vi "Subvi Email Settings.vi"() -> ()   [LabVIEW 2012]
uses:
  ProSCI Global.vi
panel:
  in  "AttachImage":bool
  in  "Carrier":string(combo)="@message.alltel.com"
  in  "Continue":bool
  in  "Cellphone Number":string
  in  "SMSMe":bool
  in  "NotifyNum":u32=5 min=5 max=10000 step=5
  in  "EmailMe":bool
  in  "CaseID":string
  # "Sequence Progress Notification"
  # "Notify through"
  # "Attach Image with Email"
  # "(* Texting may incur charges from your cellphone carrier)"
  # "sections"
  # "Notify Me on Completion and every"
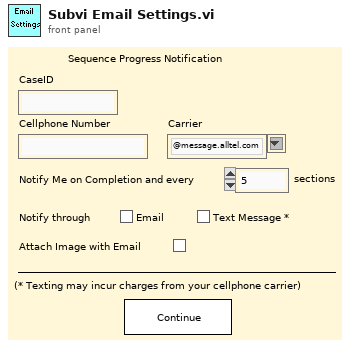
[diagram p1: front panel]
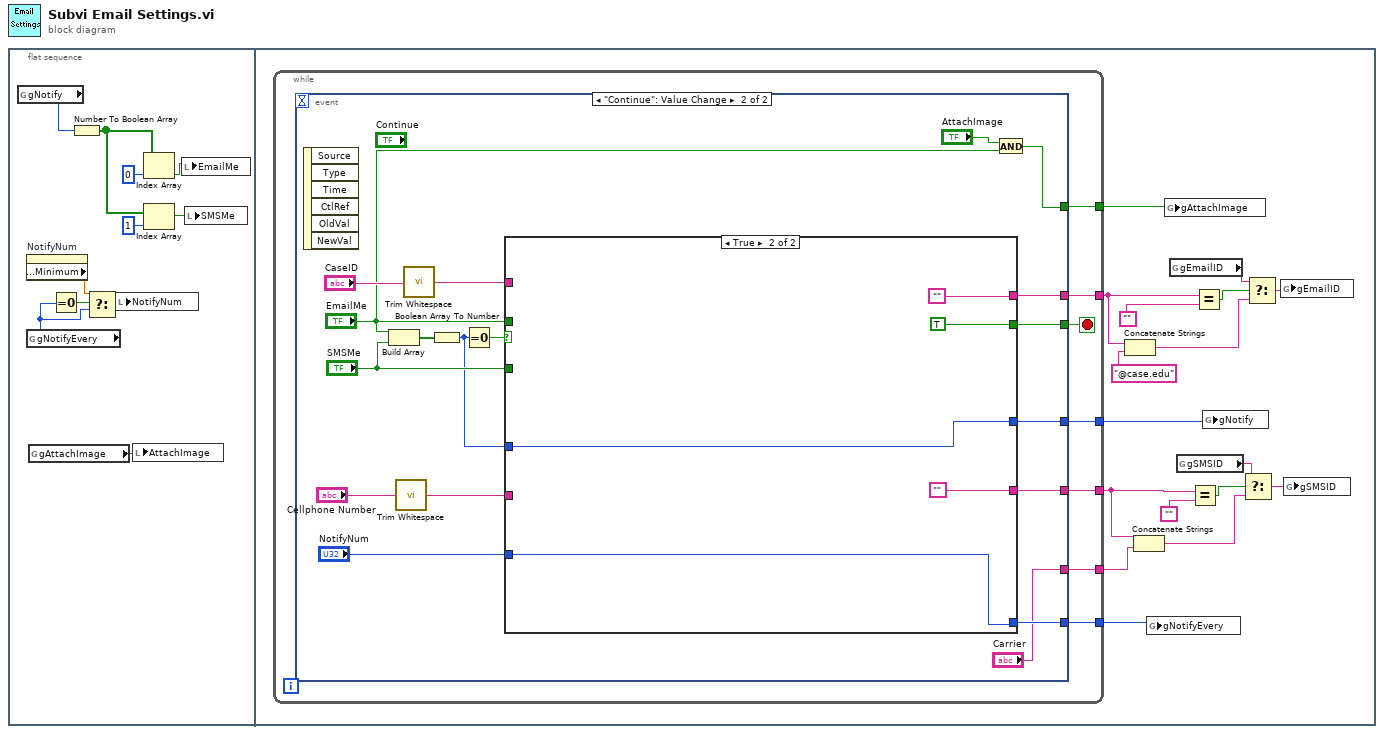
[diagram p0: block diagram]
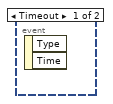
[diagram p2: hidden frame]
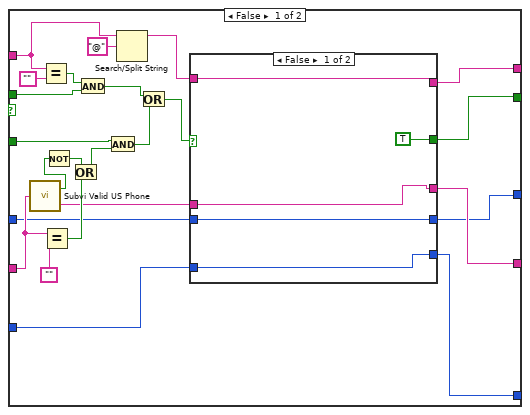
[diagram p3: hidden frame]
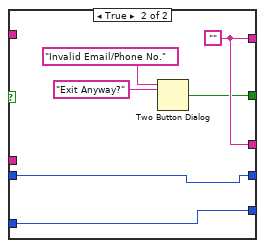
[diagram p4: hidden frame]
diagram:
  n1 = flat-sequence {
    frame #0 {
      n2 = global read "ProSCI Global.vi" "gNotify"() -> (w11:enum16{"None", "Email", "SMS", "Both"})
      n3 = property on="NotifyNum" class="DigNum (strict)"() -> ("Data Entry Limits:Minimum"=w1:dbl)  [unwired: 2 in, 2 out]
      n4 = global read "ProSCI Global.vi" "gNotifyEvery"() -> (w3:u32)
      n5 = global read "ProSCI Global.vi" "gAttachImage"() -> (w5:bool)
      n6 = Equal To 0?(x=w3) -> (x = 0?=w4:bool)
      n7 = Number To Boolean Array(number=w11) -> (Boolean array=w8:bool[])
      n8 = Select(t=w1, s=w4, f=w3) -> (s? t:f=w2:dbl)
      n9 = local write "NotifyNum"(w2) -> ()
      n10 = local write "AttachImage"(w5) -> ()
      n11 = Index Array(array=w8, index=0) -> (element=w7:bool)
      n12 = Index Array(array=w8, index=1) -> (element=w6:bool)
      n13 = local write "EmailMe"(w7) -> ()
      n14 = local write "SMSMe"(w6) -> ()
    }
    frame #1 {
      n15 = while {
        tunnel: [w34] -> w27
        tunnel: [w33] -> w22
        tunnel: [w32] -> w15
        tunnel: [w31] -> w14
        tunnel: [w30] -> w13
        tunnel: [w29] -> w12
        stop <- w35 stop-if-true
        n16 = event shown="[1] \"Continue\": Value Change" {
          selector: _ -> [_ _]
          dyn-events: _ -> [_ _]
          timeout: _ -> [_ _]
          tunnel: [_ w52] -> w35
          tunnel: [_ w48] -> w34
          tunnel: [_ w44] -> w33
          tunnel: [_ w43] -> w32
          tunnel: [_ w40] -> w31
          tunnel: [_ "Carrier"] -> w30
          tunnel: [_ w36] -> w29
          event Timeout {
            n17 = event-data() -> ()  [unwired: 3 out]
          }
          event "Continue": Value Change {
            n18 = event-data() -> ()  [unwired: 7 out]
            n19 = Build Array("EmailMe", "SMSMe") -> (w53:bool[])
            n20 = call <vilib>:"Trim Whitespace.vi"("string"="Cellphone Number") -> ("trimmed string"=w46:string)  [unwired: 1 in]
            n21 = call <vilib>:"Trim Whitespace.vi"("string"="CaseID") -> ("trimmed string"=w50:string)  [unwired: 1 in]
            n22 = Boolean Array To Number(Boolean array=w53) -> (number=w42:u32)
            n23 = Equal To 0?(x=w42) -> (x = 0?=w49:bool)
            n24 = case shown="True" w49 {
              tunnel: [w62 TRUE] -> w52
              tunnel: w50 -> [w76 _]
              tunnel: [w61 ""] -> w48
              tunnel: w46 -> [w70 _]
              tunnel: "EmailMe" -> [w72 _]
              tunnel: "SMSMe" -> [w71 _]
              tunnel: [w60 ""] -> w44
              tunnel: [w57 w89] -> w43
              tunnel: w42 -> [w56 w89]
              tunnel: "NotifyNum" -> [w55 w90]
              tunnel: [w54 w90] -> w40
              frame False {
                n25 = call "Subvi Valid US Phone.vi"("PhNumString"=w70) -> ("Is Valid"=w68:bool, "Valid Number"=w58:string)
                n26 = Equal?(x=w76, y="") -> (x = y?=w73:bool)
                n27 = Equal?(x=w70, y="") -> (x = y?=w67:bool)
                n28 = Not(x=w68) -> (.not. x?=w69:bool)
                n29 = Or(x=w69, y=w67) -> (x .or. y?=w66:bool)
                n30 = And(x=w73, y=w72) -> (x .and. y?=w65:bool)
                n31 = And(x=w71, y=w66) -> (x .and. y?=w64:bool)
                n32 = Search/Split String(string=w76, search string/char (-)="@") -> (substring before match=w59:string)  [unwired: 3 out]
                n33 = Or(x=w65, y=w64) -> (x .or. y?=w63:bool)
                n34 = case shown="False" w63 {
                  tunnel: [TRUE ("T button?") w85] -> w62
                  tunnel: [w81 w86] -> w61
                  tunnel: [w80 w86] -> w60
                  tunnel: w59 -> [w81 _]
                  tunnel: w58 -> [w80 _]
                  tunnel: [w79 w84] -> w57
                  tunnel: w56 -> [w79 w84]
                  tunnel: w55 -> [w78 w83]
                  tunnel: [w78 w83] -> w54
                  frame False {
                  }
                  frame True {
                    w86 = ""
                    n35 = Two Button Dialog(message="Invalid Email/Phone No.", 2:"Exit Anyway?" ("T button name (\"OK\")")) -> (T button?=w85:bool)  [unwired: 1 out]
                  }
                }
              }
              frame True {
              }
            }
            n36 = And(x="AttachImage", y="EmailMe") -> (x .and. y?=w36:bool)
          }
        }
      }
      n37 = Concatenate Strings(w27, "@case.edu") -> (w25:string)
      n38 = Concatenate Strings(w22, w13) -> (w23:string)
      n39 = global write "ProSCI Global.vi" "gNotifyEvery"(w14) -> ()
      n40 = global write "ProSCI Global.vi" "gAttachImage"(w12) -> ()
      n41 = global read "ProSCI Global.vi" "gEmailID"() -> (w17:string)
      n42 = global read "ProSCI Global.vi" "gSMSID"() -> (w16:string)
      n43 = Equal?(x=w22, y="") -> (x = y?=w24:bool)
      n44 = Equal?(x=w27, y="") -> (x = y?=w28:bool)
      n45 = global write "ProSCI Global.vi" "gNotify"(w15) -> ()
      n46 = Select(t=w16, s=w24, f=w23) -> (s? t:f=w20:string)
      n47 = Select(t=w17, s=w28, f=w25) -> (s? t:f=w21:string)
      n48 = global write "ProSCI Global.vi" "gEmailID"(w21) -> ()
      n49 = global write "ProSCI Global.vi" "gSMSID"(w20) -> ()
    }
  }
